vi "Testing 1SPC to 16xU32 conversion.vi"() -> ()   [LabVIEW 2015]
uses:
  <instrlib>/_niInstr/DSP/v1/Shared/Public/IQ Data.ctl
  <instrlib>/_niInstr/Basic Elements/v1/FPGA/Private/Count Down U16.vi
  <instrlib>/_niInstr/Basic Elements/v1/FPGA/Private/Count Up U16.vi
  <instrlib>/_niInstr/Basic Elements/v1/FPGA/Private/Count Up U32.vi
  DDC_7976R_v1.lvlib
  <vilib>/Analysis/NI_AALBase.lvlib
  <instrlib>/_niInstr/Basic Elements/v1/FPGA/niInstr Basic Elements v1 FPGA.lvlib
  <instrlib>/_niInstr/DSP/v1/Shared/niInstr DSP v1 Shared.lvlib
panel:
  out "Numeric Control 2":i32
  out "Waveform Chart":u8(graph)
  in  "data 2":T1
  out "ratio (16?)":dbl
  out "cntr.1SPC-IQ":u32
  out "cntr.16xU32":u32
  out "appended array":dbl[][](graph)
  out "double precision float":dbl
  out "*(type *) &x":fxp<+/-,18,1> format="%.18g"
  out "Numeric Control":u32
  in  "data":T1
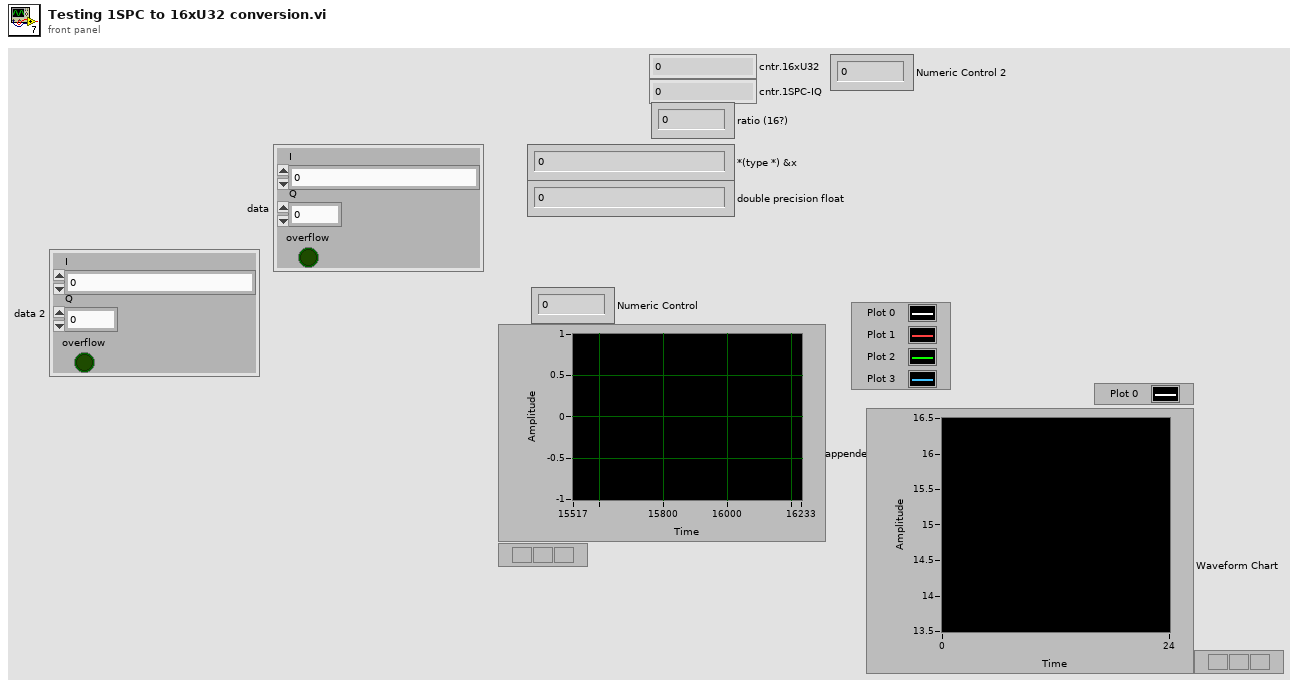
[diagram p1: front panel]
types:
  T1 = typedef "niInstr DSP v1 Shared.lvlib/IQ Data.ctl" = cluster{"I":fxp<+/-,18,1>, "Q":fxp<+/-,18,1>, "overflow":bool}
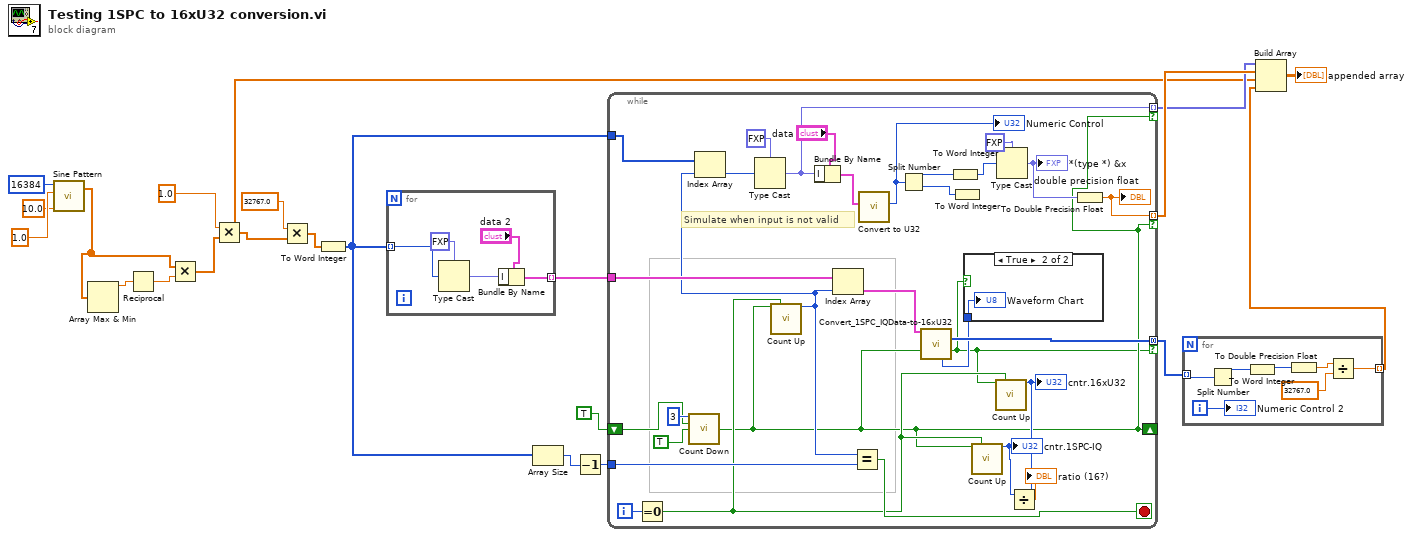
[diagram p0: block diagram]
diagram:
  n1 = call <vilib>:"Sine Pattern.vi"("cycles"=10.0, "amplitude"=1.0 ("standard deviation"), "samples"=16384) -> ("Sinusoidal Pattern"=w14:dbl[])  [unwired: 1 in, 1 out]
  n2 = Array Max & Min(array=w14) -> (max value=w15:dbl)  [unwired: 3 out]
  n3 = Reciprocal(x=w15) -> (1/x=w13:dbl)
  n4 = Multiply(x=w14, y=w13) -> (x*y=w12:dbl[])
  n5 = Multiply(x=1.0, y=w12) -> (x*y=w11:dbl[])
  n6 = Multiply(x=32767.0, y=w11) -> (x*y=w9:dbl[])
  n7 = To Word Integer(number=w9) -> (16bit integer=w1:i16[])
  n8 = for {
    tunnel: w1 -> [w23] mode=indexing
    tunnel: [w22] -> w2 mode=indexing
    n9 = Type Cast(type=fxp<+/-,18,1> 0.0 ("I"), x=w23) -> (*(type *) &x=w26:fxp<+/-,18,1>)
    n10 = Bundle By Name(cluster="data 2", "I"=w26) -> (w22:T1)
  }
  n11 = Array Size(array=w1) -> (size(s)=w4:i32)
  n12 = Decrement(x=w4) -> (x-1=w3:i32)
  n13 = while {
    tunnel: [w48] -> w20 mode=indexing if=w29
    tunnel: [w47] -> w18 mode=indexing if=w29
    tunnel: [w45] -> w7 mode=concatenating if=w27
    tunnel: w2 -> [w38]
    shift-right: [w29] -> _
    shift-left: TRUE -> [w37]
    tunnel: w3 -> [w35]
    tunnel: w1 -> [w32]
    i -> [w44]
    stop <- w36 stop-if-true
    # "Simulate when input is not valid"
    n14 = Equal To 0?(x=w44) -> (x = 0?=w34:bool)
    n15 = call-poly <instrlib>:"Count Down.vi"("count in"=u16 3, "load"=w37, "decrement"=TRUE) -> ("terminal count"=w29:bool)  [unwired: 11 in, 1 out]
    n16 = call-poly <instrlib>:"Count Up.vi"("increment"=w29, "reset"=w34) -> ("count out"=w31:u16)  [unwired: 13 in]
    n17 = Index Array(array=w32, index=w31) -> (element=w30:i16)
    n18 = Type Cast(type=fxp<+/-,18,1> 0.0 ("I"), x=w30) -> (*(type *) &x=w47:fxp<+/-,18,1>)
    n19 = Bundle By Name(cluster="data", "I"=w47) -> (w46:T1)
    n20 = Index Array(array=w38, index=w31) -> (element=w33:T1)
    n21 = Equal?(x=w31, y=w35) -> (x = y?=w36:bool)
    n22 = call "Convert to U32.vi"("IQData in"=w46) -> ("U32 out"=w56:u32)  [unwired: 8 in, 2 out]
    "Numeric Control" <- w56
    n23 = Split Number(x=w56) -> (hi(x)=w55:u16, lo(x)=w54:u16)
    n24 = call "Convert_1SPC_IQData-to-16xU32.vi"("1SPC-IQ in"=w33, "Input valid"=w29) -> ("16xU32"=w45:u32[], "Output valid"=w27:bool, "count out"=w28:u8)  [unwired: 11 in]
    n25 = To Word Integer(number=w55) -> (16bit integer=w53:i16)
    n26 = To Word Integer(number=w54) -> ()  [unwired: 1 out]
    n27 = case shown="True" w27 {
      tunnel: w28 -> [_ w57]
      frame False {
      }
      frame True {
        "Waveform Chart" <- w57
      }
    }
    n28 = call-poly <instrlib>:"Count Up.vi"("increment"=w29, "reset"=w34) -> ("count out"=w43:u32)  [unwired: 13 in]
    "cntr.1SPC-IQ" <- w43
    n29 = call-poly <instrlib>:"Count Up.vi"("increment"=w27, "reset"=w34) -> ("count out"=w42:u32)  [unwired: 13 in]
    "cntr.16xU32" <- w42
    n30 = Type Cast(type=fxp<+/-,18,1> 0.0 ("I"), x=w53) -> (*(type *) &x=w51:fxp<+/-,18,1>)
    "*(type *) &x" <- w51
    n31 = Divide(x=w43, y=w42) -> (x/y=→"ratio (16?)":dbl)
    n32 = To Double Precision Float(number=w51) -> (double precision float=w48:dbl)
    "double precision float" <- w48
  }
  n33 = for {
    tunnel: w7 -> [w64] mode=indexing
    tunnel: [w59] -> w6 mode=indexing
    i -> [w58]
    n34 = Split Number(x=w64) -> (hi(x)=w63:u16)  [unwired: 1 out]
    n35 = To Word Integer(number=w63) -> (16bit integer=w60:i16)
    n36 = To Double Precision Float(number=w60) -> (double precision float=w62:dbl)
    n37 = Divide(x=w62, y=32767.0) -> (x/y=w59:dbl)
    "Numeric Control 2" <- w58
  }
  n38 = Build Array(w18, w20, w11, w6) -> (→"appended array":dbl[][])
